vi "TestGenerator.vi"(4 "Reinit":bool, 6 "Time":u32, 11 "Test":T1) -> (0 "Done":bool, 1 "Intentionally Fail":bool, 2 "Turn":dbl, 3 "Speed":dbl)   [LabVIEW 2020]
uses:
  Tests.ctl
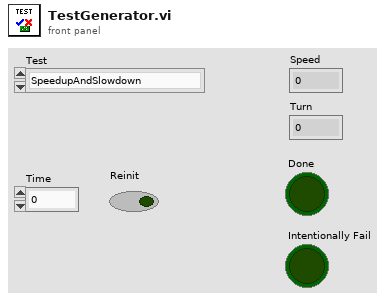
[diagram p1: front panel]
types:
  T1 = typedef "Tests.ctl" = enum16{"SpeedupAndSlowdown", "IntentionalFailure", "Figure8", "Turn360", "DriveStraightAt60", "BackInParking", "AvoidObstacle", "LaneChange", "DoNothing"}
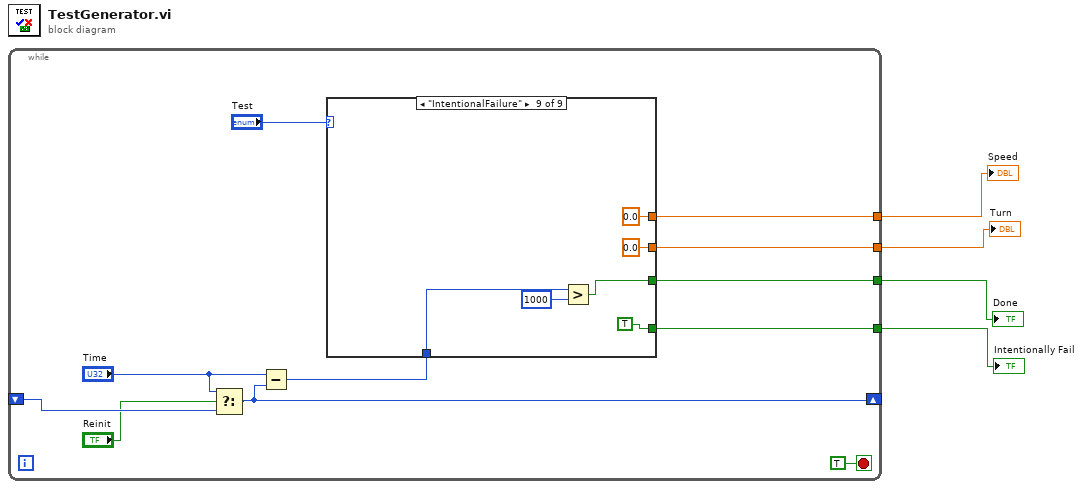
[diagram p0: block diagram]
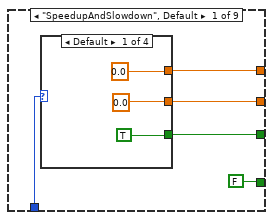
[diagram p2: hidden frame]
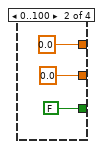
[diagram p3: hidden frame]
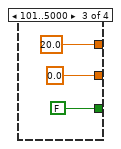
[diagram p4: hidden frame]
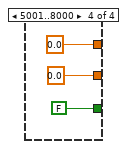
[diagram p5: hidden frame]
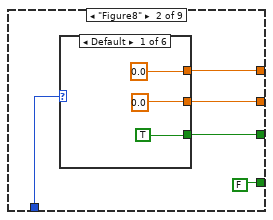
[diagram p6: hidden frame]
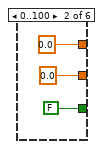
[diagram p7: hidden frame]
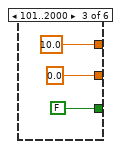
[diagram p8: hidden frame]
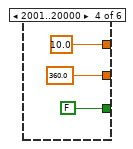
[diagram p9: hidden frame]
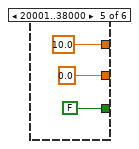
[diagram p10: hidden frame]
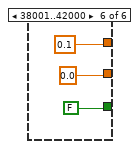
[diagram p11: hidden frame]
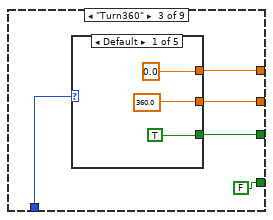
[diagram p12: hidden frame]
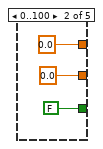
[diagram p13: hidden frame]
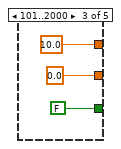
[diagram p14: hidden frame]
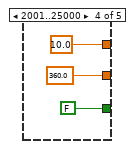
[diagram p15: hidden frame]
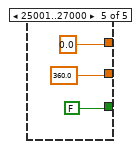
[diagram p16: hidden frame]
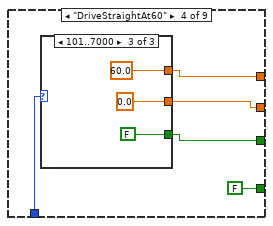
[diagram p17: hidden frame]
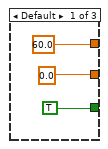
[diagram p18: hidden frame]
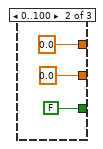
[diagram p19: hidden frame]
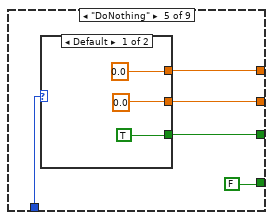
[diagram p20: hidden frame]
diagram:
  n1 = while {
    shift-right: [w13] -> _
    shift-left: _ -> [w15]
    tunnel: [w8] -> w4
    tunnel: [w7] -> w3
    tunnel: [w6] -> w2
    tunnel: [w5] -> w1
    stop <- TRUE stop-if-true
    n2 = Select(t="Time", s="Reinit", f=w15) -> (s? t:f=w13:u32)
    n3 = Subtract(x="Time", y=w13) -> (x-y=w9:u32)
    n4 = case shown="\"IntentionalFailure\"" "Test" {
      tunnel: w9 -> [w20 w37 w60 w80 w94 w105 w128 w157 w176]
      tunnel: [w19 w36 w57 w79 w93 w104 w127 w156 0.0 ("Speed")] -> w8
      tunnel: [w18 w35 w58 w78 w92 w103 w126 w155 0.0 ("Turn")] -> w7
      tunnel: [w17 w34 w59 w77 w91 w102 w125 w154 w174] -> w6
      tunnel: [FALSE ("Done") FALSE ("Done") FALSE ("Done") FALSE ("Done") FALSE ("Done") FALSE ("Done") FALSE ("Done") FALSE ("Done") TRUE ("Done")] -> w5
      frame "SpeedupAndSlowdown", Default {
        n5 = case shown="Default" w20 {
          tunnel: [0.0 ("Speed") 0.0 ("Speed") 20.0 ("Speed") 0.0 ("Speed")] -> w19
          tunnel: [0.0 ("Turn") 0.0 ("Turn") 0.0 ("Turn") 0.0 ("Turn")] -> w18
          tunnel: [TRUE ("Done") FALSE ("Done") FALSE ("Done") FALSE ("Done")] -> w17
          frame Default {
          }
          frame 0..100 {
          }
          frame 101..5000 {
          }
          frame 5001..8000 {
          }
        }
      }
      frame "Figure8" {
        n6 = case shown="Default" w37 {
          tunnel: [0.0 ("Speed") 0.0 ("Speed") 10.0 ("Speed") 10.0 ("Speed") 10.0 ("Speed") 0.1 ("Speed")] -> w36
          tunnel: [0.0 ("Turn") 0.0 ("Turn") 0.0 ("Turn") 360.0 ("Turn") 0.0 ("Turn") 0.0 ("Turn")] -> w35
          tunnel: [TRUE ("Done") FALSE ("Done") FALSE ("Done") FALSE ("Done") FALSE ("Done") FALSE ("Done")] -> w34
          frame Default {
          }
          frame 0..100 {
          }
          frame 101..2000 {
          }
          frame 2001..20000 {
          }
          frame 20001..38000 {
          }
          frame 38001..42000 {
          }
        }
      }
      frame "Turn360" {
        n7 = case shown="Default" w60 {
          tunnel: [0.0 ("Speed") 0.0 ("Speed") 10.0 ("Speed") 10.0 ("Speed") 0.0 ("Speed")] -> w57
          tunnel: [360.0 ("Turn") 0.0 ("Turn") 0.0 ("Turn") 360.0 ("Turn") 360.0 ("Turn")] -> w58
          tunnel: [TRUE ("Done") FALSE ("Done") FALSE ("Done") FALSE ("Done") FALSE ("Done")] -> w59
          frame Default {
          }
          frame 0..100 {
          }
          frame 101..2000 {
          }
          frame 2001..25000 {
          }
          frame 25001..27000 {
          }
        }
      }
      frame "DriveStraightAt60" {
        n8 = case shown="101..7000" w80 {
          tunnel: [60.0 ("Speed") 0.0 ("Speed") 60.0 ("Speed")] -> w79
          tunnel: [0.0 ("Turn") 0.0 ("Turn") 0.0 ("Turn")] -> w78
          tunnel: [TRUE ("Done") FALSE ("Done") FALSE ("Done")] -> w77
          frame Default {
          }
          frame 0..100 {
          }
          frame 101..7000 {
          }
        }
      }
      frame "DoNothing" {
        n9 = case shown="Default" w94 {
          tunnel: [0.0 ("Speed") 0.0 ("Speed")] -> w93
          tunnel: [0.0 ("Turn") 0.0 ("Turn")] -> w92
          tunnel: [TRUE ("Done") FALSE ("Done")] -> w91
          frame Default {
          }
          frame 0..1000 {
          }
        }
      }
      frame "BackInParking" {
        n10 = case shown="7001..8000" w105 {
          tunnel: [0.0 ("Speed") 0.0 ("Speed") 5.0 ("Speed") 0.0 ("Speed") -1.0 ("Speed") 0.0 ("Speed")] -> w104
          tunnel: [-90.0 ("Turn") 0.0 ("Turn") 0.0 ("Turn") 0.0 ("Turn") -90.0 ("Turn") -90.0 ("Turn")] -> w103
          tunnel: [TRUE ("Done") FALSE ("Done") FALSE ("Done") FALSE ("Done") FALSE ("Done") FALSE ("Done")] -> w102
          frame Default {
          }
          frame 0..100 {
          }
          frame 101..1000 {
          }
          frame 1001..2000 {
          }
          frame 2001..7000 {
          }
          frame 7001..8000 {
          }
        }
      }
      frame "AvoidObstacle" {
        n11 = case shown="Default" w128 {
          tunnel: [60.0 ("Speed") 0.0 ("Speed") 60.0 ("Speed") 60.0 ("Speed") 60.0 ("Speed") 60.0 ("Speed") 60.0 ("Speed") 60.0 ("Speed")] -> w127
          tunnel: [0.0 ("Turn") 0.0 ("Turn") 0.0 ("Turn") -10.0 ("Turn") 0.0 ("Turn") 10.0 ("Turn") 0.0 ("Turn") 0.0 ("Turn")] -> w126
          tunnel: [TRUE ("Done") FALSE ("Done") FALSE ("Done") FALSE ("Done") FALSE ("Done") FALSE ("Done") FALSE ("Done") FALSE ("Done")] -> w125
          frame Default {
          }
          frame 0..100 {
          }
          frame 101..5000 {
          }
          frame 5001..6000 {
          }
          frame 6001..7000 {
          }
          frame 7001..8000 {
          }
          frame 8001..9000 {
          }
          frame 9001..10000 {
          }
        }
      }
      frame "LaneChange" {
        n12 = case shown="Default" w157 {
          tunnel: [60.0 ("Speed") 0.0 ("Speed") 60.0 ("Speed") 60.0 ("Speed") 60.0 ("Speed")] -> w156
          tunnel: [0.0 ("Turn") 0.0 ("Turn") 0.0 ("Turn") -10.0 ("Turn") 0.0 ("Turn")] -> w155
          tunnel: [TRUE ("Done") FALSE ("Done") FALSE ("Done") FALSE ("Done") FALSE ("Done")] -> w154
          frame Default {
          }
          frame 0..100 {
          }
          frame 101..5000 {
          }
          frame 5001..6000 {
          }
          frame 6001..7000 {
          }
        }
      }
      frame "IntentionalFailure" {
        n13 = Greater?(x=w176, y=u32 1000) -> (0:w174:bool)
      }
    }
  }
  "Speed" <- w4
  "Turn" <- w3
  "Done" <- w2
  "Intentionally Fail" <- w1
